vi "write_ui_stop_notifier.vi"(8 "error in (no error)":errorcluster, 10 "stop_ui_notifier":refnum<user-event>, 11 "panel in":refnum<class "panel.lvclass">) -> (0 "error out":errorcluster, 3 "panel out":refnum<class "panel.lvclass">)   [LabVIEW 2015, in "panel.lvclass"]
uses:
  panel.lvclass
  panel.lvclass/panel.ctl
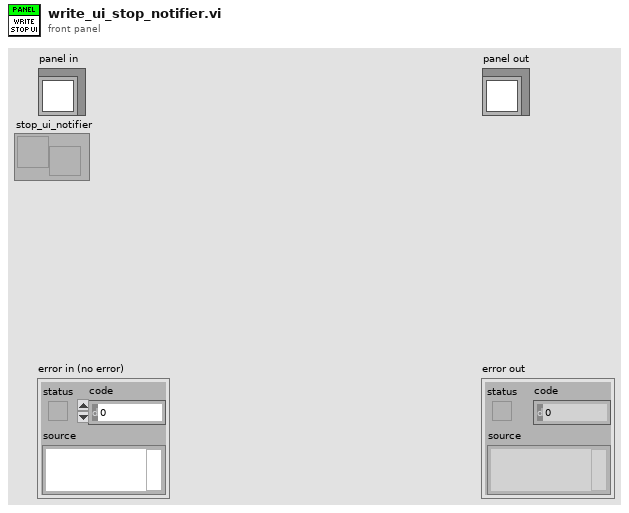
[diagram p1: front panel]
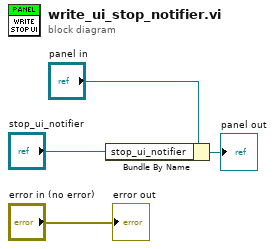
[diagram p0: block diagram]
diagram:
  n1 = Bundle By Name(cluster="panel in", "stop_ui_notifier"="stop_ui_notifier") -> (→"panel out":refnum<class "panel.lvclass">)
  "error out" <- "error in (no error)"
